vi "Configure Interpolation [I] Core.vi"(8 "error in (no error)":errorcluster, 10 "interpolation":i32(ring)=1 items=["No Interpolation"=1, "sin(x)/x"=2, "Linear Interpolation"=3], 11 "IVI_Scope in":refnum<class "IVI_Scope.lvclass">) -> (0 "error out":errorcluster, 3 "IVI_Scope out":refnum<class "IVI_Scope.lvclass">)   [LabVIEW 2016, in "IVI_Scope.lvlib" / "IVI_Scope.lvclass"]
doc: "This VI configures the interpolation method the oscilloscope uses when it cannot sample a voltage for a point in the waveform record. \n\nNotes:\n\n(1) This VI is part of the miscellaneous [*] extension group."
uses:
  IVI_Scope.lvclass
  IVI_Scope.lvclass/IVI_Scope.ctl
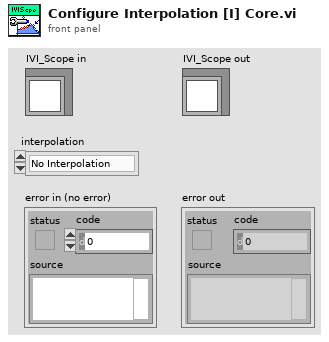
[diagram p1: front panel]
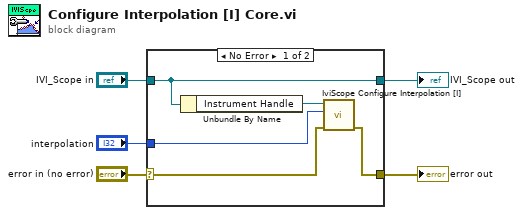
[diagram p0: block diagram]
diagram:
  n1 = case shown="No Error" "error in (no error)" {
    selector: "error in (no error)" -> [w8 w12]
    tunnel: [w7 w12] -> w4
    tunnel: [w10 w11] -> w2
    tunnel: "IVI_Scope in" -> [w10 w11]
    tunnel: "interpolation" -> [w6 _]
    frame No Error {
      n2 = Unbundle By Name(w10) -> ("Instrument Handle"=w9:refnum<k15>)
      n3 = call <vilib>:"IviScope Configure Interpolation [I].vi"("error in (no error)"=w8, "interpolation"=w6, "instrument handle"=w9) -> ("error out"=w7:errorcluster)  [unwired: 7 in, 1 out]
    }
    frame Error {
    }
  }
  "error out" <- w4
  "IVI_Scope out" <- w2
